vi "Prueba_tipos.vi"() -> ()   [LabVIEW 2015]
panel:
  in  "index":i32=1
  out "Data Entry Limits:Minimum":dbl
  out "Data Entry Limits:Maximum":dbl
  out "error out":errorcluster
  in  "String":string
  out "Label.Text":string
  out "Description 2":string
  out "Description":string
  out "Control Index":i32
  out "size(s)":i32
  out "Name":string
  out "Get Control Index by Name":i32
  out "element":refnum<vi>
  in  "vi path":path=path "C:/Users/Usuario/Desktop/DICTINO/PROYECTOS/rip-labview-server-integrado/rip-labview-server/Private/JiLTestOK.vi"
  out "Numeric":dbl
  out "Control Value:Get All":cluster{"Name":string, "Variant Data":variant}[](array[cluster])
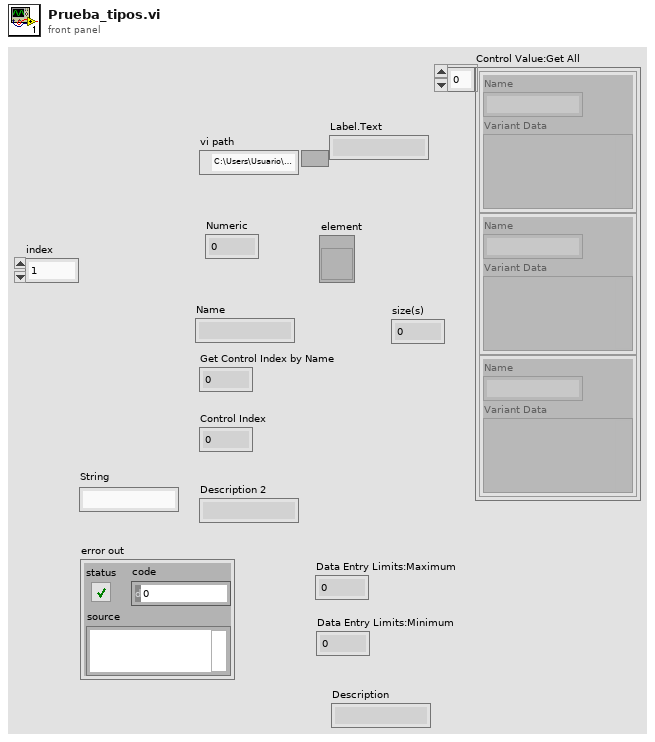
[diagram p1: front panel]
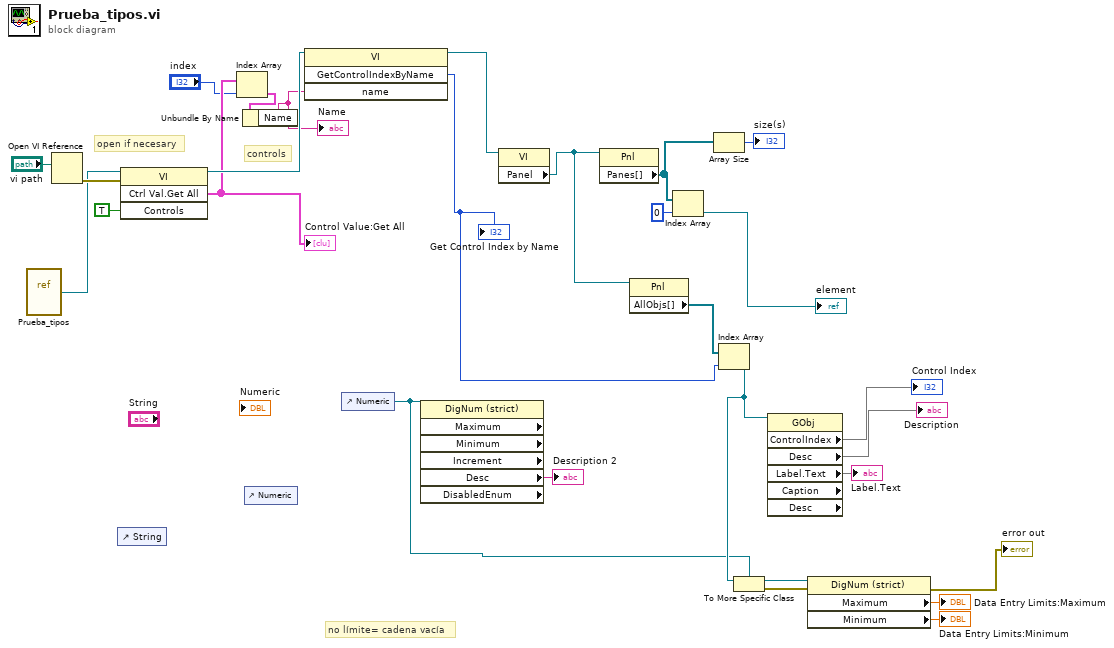
[diagram p0: block diagram]
diagram:
  # "no límite= cadena vacía"
  # "controls"
  # "open if necesary"
  n1 = vi-ref "Prueba_tipos.vi"() -> (w19:refnum<vi>)
  n2 = Open VI Reference(vi path="vi path") -> (error out=w26:errorcluster)  [unwired: 2 in, 4 out]
  n3 = control-ref of="String"() -> ()  [unwired: 1 out]
  n4 = invoke class="VI" method="Ctrl Val.Get All"(reference=w19, error in=w26, "Controls"=TRUE) -> (reference out=w28:refnum<vi>, "Get All Control Values Variant"=w25:cluster{"Name":string, "Variant Data":variant}[])  [unwired: 1 in, 2 out]
  "Control Value:Get All" <- w25
  n5 = Index Array(array=w25, index="index") -> (element=w23:cluster{"Name":string, "Variant Data":variant})
  n6 = Unbundle By Name(w23) -> ("Name"=w22:string)
  "Name" <- w22
  n7 = control-ref of="Numeric"() -> ()  [unwired: 1 out]
  n8 = invoke class="VI" method="GetControlIndexByName"(reference=w28, "name"=w22) -> (reference out=w20:refnum<vi>, "GetControlIndexByName"=w13:i32)  [unwired: 2 in, 2 out]
  "Get Control Index by Name" <- w13
  n9 = control-ref of="Numeric"() -> (w6:refnum<vi>)
  n10 = property class="DigNum (strict)" props=["Maximum", "Minimum", "Increment", "Desc", "DisabledEnum"](reference=w6) -> ("Desc"=→"Description 2":string)  [unwired: 1 in, 6 out]
  n11 = property class="VI"(reference=w20) -> ("Panel"=w9:refnum<vi>)  [unwired: 1 in, 2 out]
  n12 = property class="Pnl"(reference=w9) -> ("Panes[]"=w18:refnum<vi>[])  [unwired: 1 in, 2 out]
  n13 = property class="Pnl"(reference=w9) -> ("AllObjs[]"=w14:refnum<vi>[])  [unwired: 1 in, 2 out]
  n14 = Index Array(array=w18, index=0) -> (element=→"element":refnum<vi>)
  n15 = Array Size(array=w18) -> (size(s)=→"size(s)":i32)
  n16 = Index Array(array=w14, index=w13) -> (element=w7:refnum<vi>)
  n17 = To More Specific Class(target class=w6, reference=w7) -> (specific class reference=w5:refnum<vi>, error out=w2:errorcluster)  [unwired: 1 in]
  n18 = property class="GObj" props=["ControlIndex", "Desc", "Label", "Text", "Caption", "Desc"](reference=w7) -> ("ControlIndex"=→"Control Index", "Desc"=→"Description", "Label.Text"=→"Label.Text")  [unwired: 1 in, 4 out]
  n19 = property class="DigNum (strict)"(reference=w5, error in=w2) -> (error out=→"error out":errorcluster, "Maximum"=→"Data Entry Limits:Maximum":dbl, "Minimum"=→"Data Entry Limits:Minimum":dbl)  [unwired: 1 out]
